vi "ErrorHandling.CloseErrorHandler.vi"(8 "ErrorIn":errorcluster) -> (0 "ErrorOut":errorcluster)   [LabVIEW 2016, in "ErrorHandling.lvclass"]
uses:
  ErrorHandling.lvclass
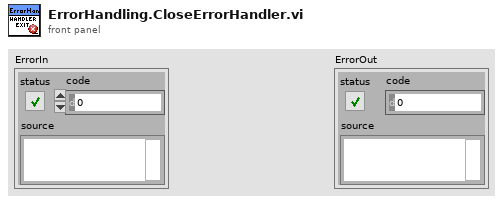
[diagram p1: front panel]
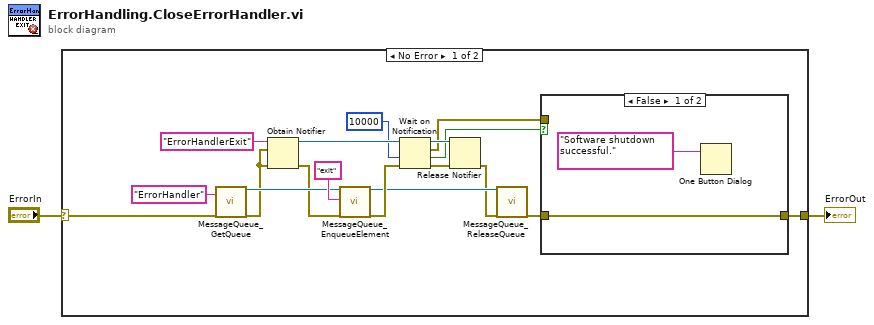
[diagram p0: block diagram]
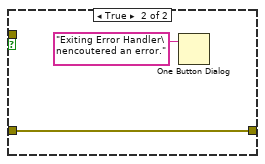
[diagram p2: hidden frame]
diagram:
  n1 = case shown="No Error" "ErrorIn" {
    selector: "ErrorIn" -> [w17 w25]
    tunnel: [w3 w25] -> w2
    frame No Error {
      n2 = call "MessageQueue_GetQueue.vi"("Name"="ErrorHandler", "ErrorIn"=w17) -> ("QueueOut"=w18:refnum<queue>, "ErrorOut"=w7:errorcluster)  [unwired: 15 in, 1 out]
      n3 = Obtain Notifier(name (unnamed)="ErrorHandlerExit", notification data type=w7, error in (no error)=w7) -> (notifier out=w15:refnum<notifier>, error out=w13:errorcluster)  [unwired: 1 in, 1 out]
      n4 = call "MessageQueue_EnqueueElement.vi"("QueueIn"=w18, "Message"="exit", "ErrorIn"=w13) -> ("QueueOut"=w10:refnum<queue>, "ErrorOut"=w12:errorcluster)  [unwired: 15 in]
      n5 = Wait on Notification(notifier=w15, timeout in ms (-1)=10000, error in (no error)=w12) -> (notifier out=w14:refnum<notifier>, notification=w5:errorcluster, timed out?=w6:bool, error out=w11:errorcluster)  [unwired: 1 in]
      n6 = Release Notifier(notifier=w14, error in (no error)=w11) -> (error out=w9:errorcluster)  [unwired: 1 in, 2 out]
      n7 = call "MessageQueue_ReleaseQueue.vi"("QueueIn"=w10, "ErrorIn"=w9) -> ("ErrorOut"=w4:errorcluster)  [unwired: 15 in, 2 out]
      n8 = case shown="False" w6 {
        tunnel: w5 -> [_ _]
        tunnel: w4 -> [w22 w24]
        tunnel: [w22 w24] -> w3
        frame False {
          n9 = One Button Dialog(message="Software shutdown successful.") -> ()  [unwired: 1 in, 1 out]
        }
        frame True {
          n10 = One Button Dialog(message="Exiting Error Handler\nencoutered an error.") -> ()  [unwired: 1 in, 1 out]
        }
      }
    }
    frame Error {
    }
  }
  "ErrorOut" <- w2
